vi "Write Buffer 1D U64.vi"(7 "count (-1: all)":i64=-1 format="%d elements", 8 "error in (no error)":errorcluster, 9 "offset (0)":u64 format="%d bytes", 10 "src array in":u64[](array[numeric]), 11 "Buffer in":refnum<class "Buffer.lvclass">) -> (0 "error out":errorcluster, 1 "offset out":u64 format="%d bytes", 2 "src array out":u64[](array[numeric]), 3 "Buffer out":refnum<class "Buffer.lvclass">)   [LabVIEW 2017, in "DSF Core.lvlib" / "Buffer.lvclass"]
doc: "Writes <b>count</b> elements from <b>src array</b> into <b>Buffer</b> at the specified <b>offset</b>."
uses:
  Buffer.lvclass
  C:/Git/DSF/LabVIEW-Memory/Source/Classes/Pointer/Pointer.lvclass
  LabVIEW-Memory/Source/Classes/Pointer/Write 1D U64.vi
  LabVIEW-Memory/Source/Classes/Pointer/Pointer.lvclass
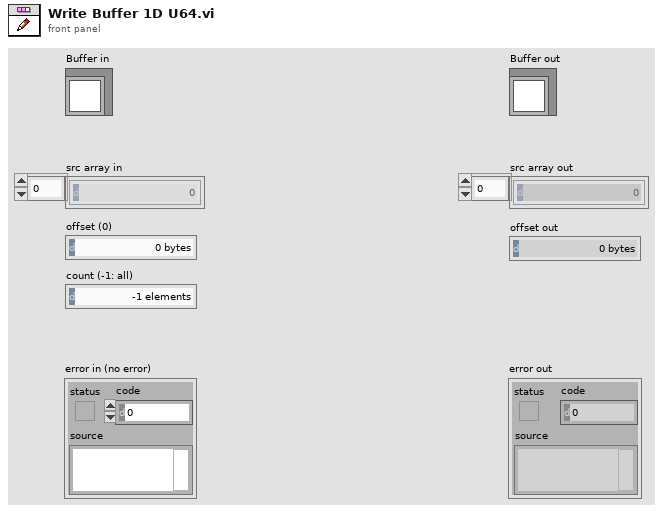
[diagram p1: front panel]
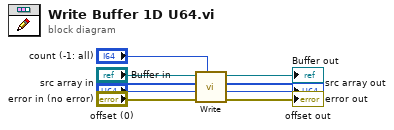
[diagram p0: block diagram]
diagram:
  n1 = call-poly "Write.vi"("count (-1: all)"="count (-1: all)", "error in (no error)"="error in (no error)", "offset (0)"="offset (0)", "buffer in"="src array in", "Pointer in"="Buffer in") -> ("error out"=→"error out":errorcluster, "offset + size"=→"offset out":u64, "buffer out"=→"src array out":u64[], "Pointer out"=→"Buffer out":refnum<class "Buffer.lvclass">)  [unwired: 3 in]
